vi "Handle Error.vi"(8 "error in (no error)":errorcluster, 11 "CS++BaseActor in":refnum<class "CS++BaseActor.lvclass">) -> (0 "error out":errorcluster, 2 "stop actor?":bool=TRUE, 3 "CS++BaseActor out":refnum<class "CS++BaseActor.lvclass">)   [LabVIEW 2012, in "CS++BaseActor.lvlib" / "CS++BaseActor.lvclass"]
doc: "(<B>Filename</B>: Actor Framework.lvlib:Actor.lvclass:Handle Error.vi)\n\nDefines how the actor handles an error that occurred while processing a message.\n\nBy default, this method does nothing except stop the actor. This method also treats error code 43 (coming from <B>error in</B>) as a sign that the actor shut down normally. In this situation, the Handle Error method does not return the error on <B>error out</B>, meaning the actor's caller will not receive it. All other error codes will be returned on <B>error out</B>.\n\nA descendant class may override this method to change this behavior."
uses:
  CS++BaseActor.lvclass
  <vilib>/ActorFramework/Actor/Actor.lvclass
  <vilib>/Utility/error.llb/DialogType.ctl
  Libraries/MessageLogger/CS++MessageLogger.lvlib
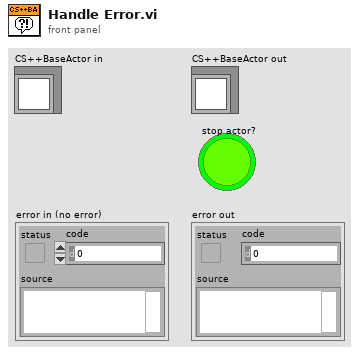
[diagram p1: front panel]
types:
  T1 = typedef "DialogType.ctl" = u16
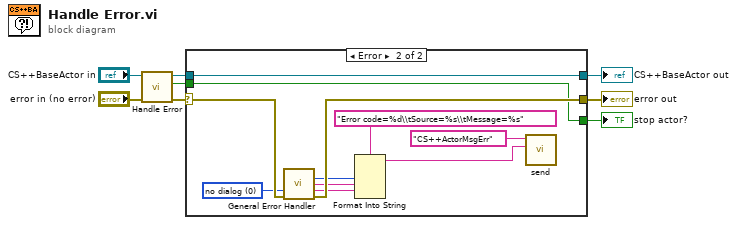
[diagram p0: block diagram]
diagram:
  n1 = call-parent "Handle Error.vi"("error in (no error)"="error in (no error)", "Actor in"="CS++BaseActor in") -> ("error out"=w6:errorcluster, "stop actor?"=w3:bool, "Actor out"=w1:refnum<class "CS++BaseActor.lvclass">)  [unwired: 7 in]
  n2 = case shown="Error" w6 {
    selector: w6 -> [w11 w21]
    tunnel: [w11 w19] -> w5
    tunnel: [w10 w18] -> w4
    tunnel: w3 -> [w10 w18]
    tunnel: [w9 w22] -> w2
    tunnel: w1 -> [w9 w22]
    frame No Error {
    }
    frame Error {
      w20 = T1 0 items=["no dialog", "OK message", "continue or stop message", "OK message + warnings", "continue/stop + warnings"] ("type of dialog (OK msg:1)")
      n3 = call <vilib>:"General Error Handler.vi"("type of dialog (OK msg:1)"=w20, "error in (no error)"=w21) -> ("code out"=w16:i32, "source out"=w15:string, "message"=w14:string, "error out"=w19:errorcluster)  [unwired: 9 in, 1 out]
      n4 = Format Into String(format string="Error code=%d\\tSource=%s\\tMessage=%s", w16, w15, w14) -> (resulting string=w12:string)  [unwired: 2 in, 1 out]
      n5 = call "send.vi"("Message Content"=w12, "Message Tag"="CS++ActorMsgErr") -> ()  [unwired: 9 in, 1 out]
    }
  }
  "CS++BaseActor out" <- w2
  "error out" <- w5
  "stop actor?" <- w4
